vi "buildTagURL.vi"(10 "LastVersion":T1, 11 "URL":string="https://svn.cim.as/svn/CIM_TM/Projects/3173 SVS - SmartVisionSystem/LV2017/trunk/LabVIEW") -> (2 "tagname":string, 3 "TagURL":string)   [LabVIEW 2017]
uses:
  <vilib>/AppBuilder/AB_API_Simple/Build Specification Version.ctl
  <vilib>/AppBuilder/AB_API_Simple/NI_App_Builder_API.lvlib
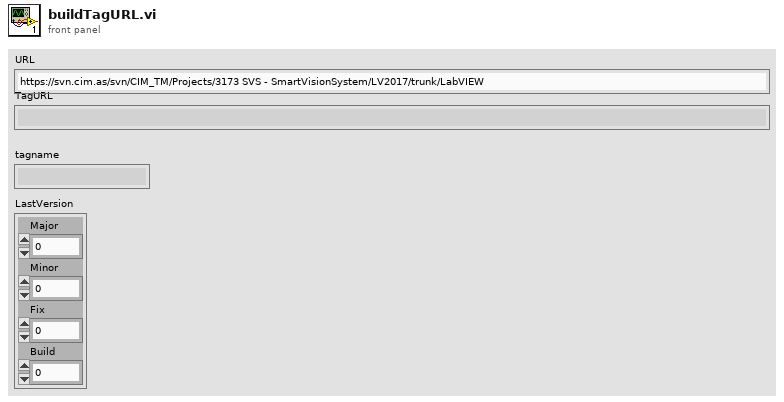
[diagram p1: front panel]
types:
  T1 = typedef "NI_App_Builder_API.lvlib/Build Specification Version.ctl" = cluster{"Major":u16, "Minor":u16, "Fix":u16, "Build":u16}
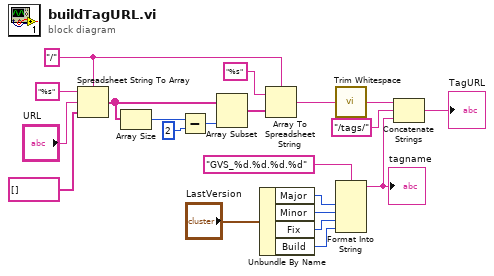
[diagram p0: block diagram]
diagram:
  w15 = "/" ("delimiter (Tab)")
  n1 = Spreadsheet String To Array(delimiter (Tab)=w15, format string="%s", spreadsheet string="URL", array type (2D Dbl)=string[] []) -> (array=w19:string[])
  n2 = Array Size(array=w19) -> (size(s)=w18:i32)
  n3 = Subtract(x=w18, y=2) -> (x-y=w16:i32)
  n4 = Array Subset(array=w19, length=w16) -> (w14:string[])  [unwired: 1 in]
  n5 = Unbundle By Name("LastVersion") -> ("Major"=w5:u16, "Minor"=w4:u16, "Fix"=w3:u16, "Build"=w2:u16)
  n6 = Array To Spreadsheet String(delimiter (Tab)=w15, array=w14, 3:"%s" ("format string")) -> (spreadsheet string=w10:string)
  n7 = call <vilib>:"Trim Whitespace.vi"("string"=w10) -> ("trimmed string"=w9:string)  [unwired: 1 in]
  n8 = Format Into String(format string="GVS_%d.%d.%d.%d", w5, w4, w3, w2) -> (resulting string=w1:string)  [unwired: 2 in, 1 out]
  "tagname" <- w1
  n9 = Concatenate Strings(w9, "/tags/" ("format string"), w1) -> (→"TagURL":string)
